vi "Periodic Log Filter Check.vi"(0 "Cross CSM Data":T2={"Name (\"\" to Use UUID)"="CSM Tiny", "Current State"="UI: Refresh Buttons", "Arguments"="", "Source Message"={"‘State"="", "’Arguments"="", "’Error"={"status"=FALSE, "code"=0, "source"=""}}, "Source Module"="<end>", "Complete(T)/Start(F)"=TRUE, "LogType"=enum."State Change", "Time Stamp"=timestamp(0 s since 1904-01-01)}, 1 "Reset?":bool, 9 "Remove Immediately? (F)":bool, 11 "Settings":T5={"threashold(#/s)"=2.0, "Check Peroid(s)"=1.0}, 12 "Level (Normal)":T1) -> (4 "Cross CSM Data Out":T2={"Name (\"\" to Use UUID)"="", "Current State"="", "Arguments"="", "Source Message"={"‘State"="", "’Arguments"="", "’Error"={"status"=FALSE, "code"=0, "source"=""}}, "Source Module"="", "Complete(T)/Start(F)"=FALSE, "LogType"=enum."State Change", "Time Stamp"=timestamp(0 s since 1904-01-01)}, 6 "Current Time":timestamp, 10 "Additional Info":string[](array[string]), 14 "Filtered Status":string[](array[string]), 15 "Filtered":bool)   [LabVIEW 2017, in "Communicable State Machine.lvlib" / "LogFilter.lvclass"]
uses:
  LogFilter.lvclass
  Typedef/_CSM_GlobalLog_MSG.ctl
  Typedef/_CSM_Response Source Message.ctl
  Typedef/_CSM_GlobalLog_MSG_TYPE.ctl
  Utility/_support/Periodic String Filter Level.ctl
  Utility/Periodic String Filter State.ctl
  Communicable State Machine.lvlib
  _Shared/CSM Shared.lvlib
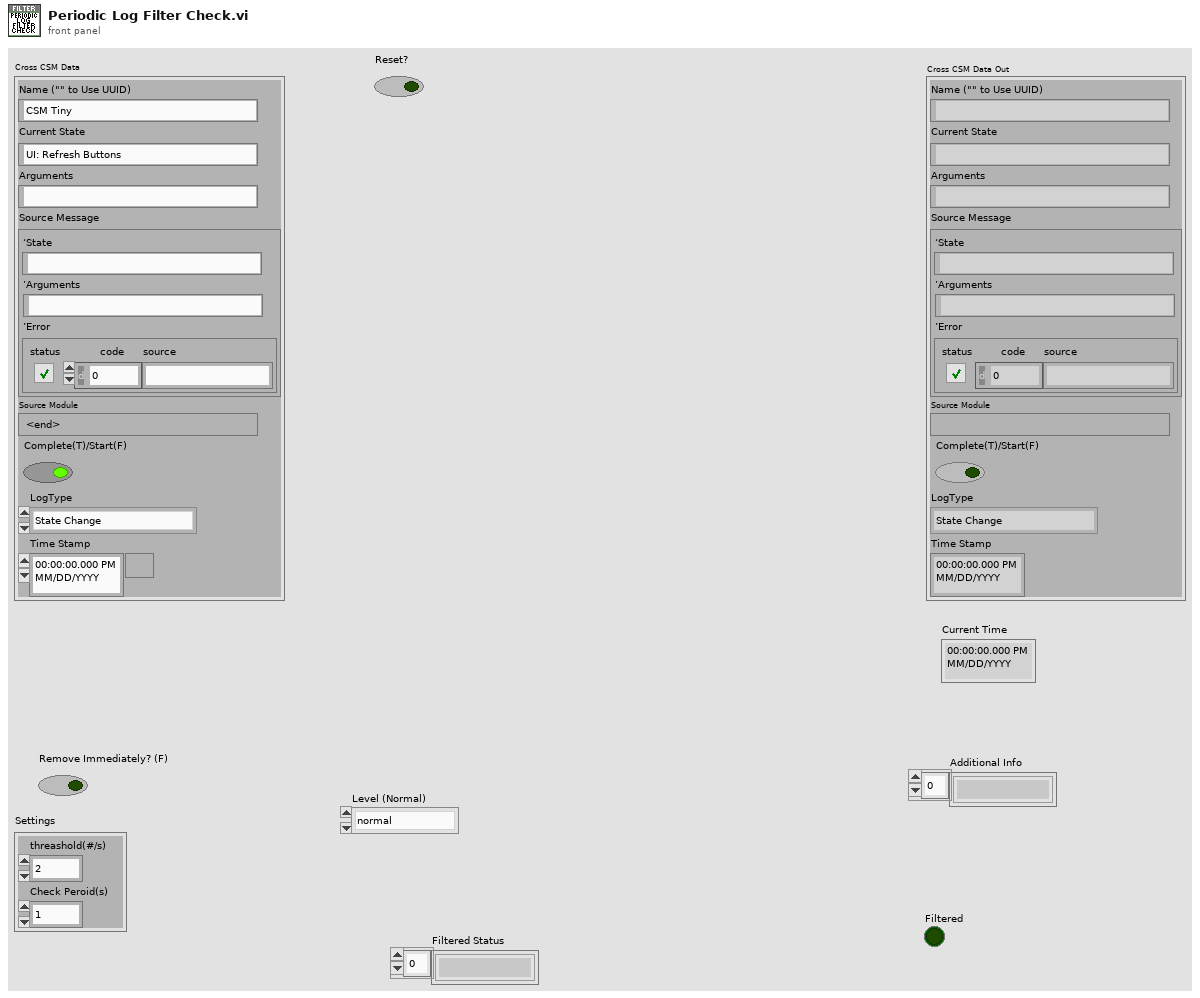
[diagram p1: front panel]
types:
  T1 = typedef "Communicable State Machine.lvlib/Periodic String Filter Level.ctl" = enum16{"normal", "L1", "L2", "L3", "L4"}
  T2 = typedef "Communicable State Machine.lvlib/_CSM_GlobalLog_MSG.ctl" = cluster{"Name (\"\" to Use UUID)":string, "Current State":string, "Arguments":string, "Source Message":T3, "Source Module":string, "Complete(T)/Start(F)":bool, "LogType":T4, "Time Stamp":timestamp}
  T3 = typedef "Communicable State Machine.lvlib/_CSM_Response Source Message.ctl" = cluster{"‘State":string, "’Arguments":string, "’Error":errorcluster}
  T4 = typedef "Communicable State Machine.lvlib/_CSM_GlobalLog_MSG_TYPE.ctl" = enum16{"User Log", "State Change", "Status", "Interrupt", "Register", "Unregister", "Error Log", "Module Created", "Module Destroyed", "Async Message", "No-Rep Async Message", "Sync Message", "AsyncMsg Complete", "SyncMsg Complete"}
  T5 = cluster{"threashold(#/s)":dbl, "Check Peroid(s)":dbl}
  T6 = typedef "Communicable State Machine.lvlib/Periodic String Filter State.ctl" = enum16{"Normal", "Remove All Filters"}
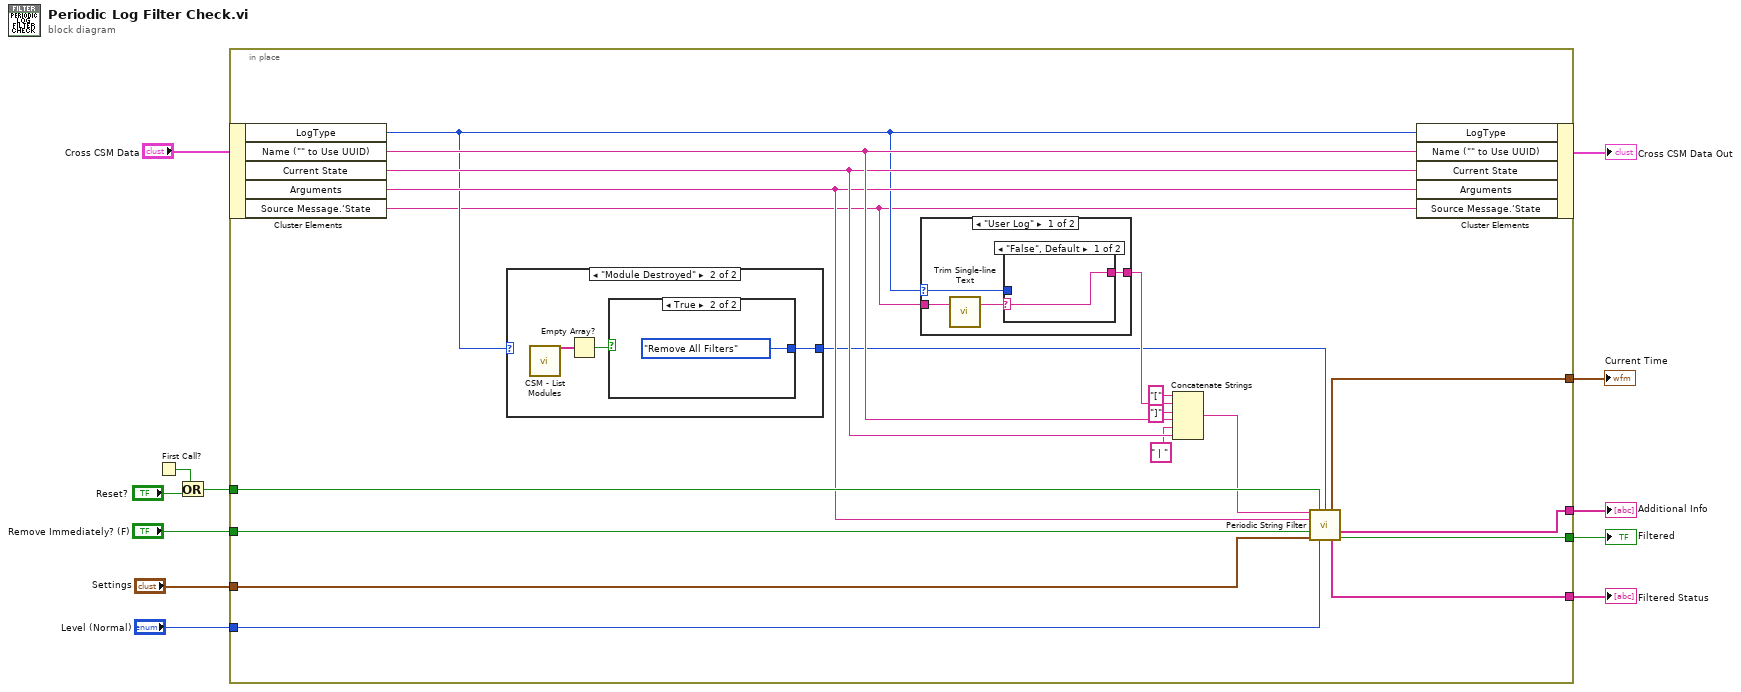
[diagram p0: block diagram]
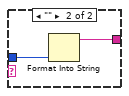
[diagram p2: hidden frame]
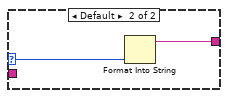
[diagram p3: hidden frame]
diagram:
  n1 = First Call?() -> (First Call?: T/F=w11:bool)
  n2 = Or(x=w11, y="Reset?") -> (x .or. y?=w9:bool)
  n3 = in-place {
    in-place-border: w9 -> [w28]
    in-place-border: [w26] -> w8
    in-place-border: "Remove Immediately? (F)" -> [w23]
    in-place-border: "Settings" -> [w22]
    in-place-border: [w21] -> w1
    in-place-border: [w20] -> w4
    in-place-border: "Level (Normal)" -> [w17]
    in-place-border: [w16] -> w2
    n4 = in-place-cluster #1("Cross CSM Data") -> ("LogType"=w15:T4, "Name (\"\" to Use UUID)"=w31:string, "Current State"=w30:string, "Arguments"=w19:string, "Source Message.‘State"=w13:string)
    n5 = case shown="\"Module Destroyed\"" w15 {
      tunnel: [_ w41] -> w14
      frame "User Log", Default {
      }
      frame "Module Destroyed" {
        n6 = call "CSM - List Modules.vi"() -> ("Module Names"=w43:string[])  [unwired: 10 in, 1 out]
        n7 = Empty Array?(array=w43) -> (empty?=w42:bool)
        n8 = case shown="True" w42 {
          tunnel: [_ Periodic_String_Filter_State."Remove All Filters" ("State")] -> w41
          frame False {
          }
          frame True {
          }
        }
      }
    }
    n9 = case shown="\"User Log\"" w15 {
      selector: w15 -> [w34 w39]
      tunnel: [w35 w40] -> w18
      tunnel: w13 -> [w33 _]
      frame "User Log" {
        n10 = call "Trim Single-line Text.vi"("single-line text"=w33) -> ("trimed text"=w32:string)  [unwired: 2 in]
        n11 = case shown="\"False\", Default" w32 {
          selector: w32 -> [w36 _]
          tunnel: [w36 w38] -> w35
          tunnel: w34 -> [_ w37]
          frame "False", Default {
          }
          frame "" {
            n12 = Format Into String(w37) -> (resulting string=w38:string)  [unwired: 3 in, 1 out]
          }
        }
      }
      frame Default {
        n13 = Format Into String(w39) -> (resulting string=w40:string)  [unwired: 3 in, 1 out]
      }
    }
    n14 = Concatenate Strings("[" ("string"), w18, "]" ("string"), w31, " | " ("string"), w30) -> (w27:string)
    n15 = call "Periodic String Filter.vi"("Input String"=w27, "Reset?"=w28, "State"=w14, "Parameter"=w19, "Remove Immediately? (F)"=w23, "Settings"=w22, "Level (Normal)"=w17) -> ("Current Time"=w16:timestamp, "Additional Info"=w20:string[], "Filtered Status"=w21:string[], "Filtered?"=w26:bool)  [unwired: 4 in, 1 out]
    n16 = in-place-cluster #1("LogType"=w15, "Name (\"\" to Use UUID)"=w31, "Current State"=w30, "Arguments"=w19, "Source Message.‘State"=w13) -> (→"Cross CSM Data Out":T2)
  }
  "Filtered" <- w8
  "Filtered Status" <- w1
  "Additional Info" <- w4
  "Current Time" <- w2
